vi "Outlook_Body_InsertPicture.vi"(7 "show Image in the Attachments? (F)":bool, 8 "error in (no error)":errorcluster, 9 "FilePath":path, 11 "Attachment Refnum (In)":refnum<k7>) -> (0 "error out":errorcluster, 1 "PathName":string, 2 "FileName":string, 3 "Attachment Refnum (Out)":refnum<k7>, 4 "DisplayName":string, 6 "Class":i32)   [LabVIEW 2014]
panel:
  out "Size":i32
  out "Position":i32
  out "Type":i32
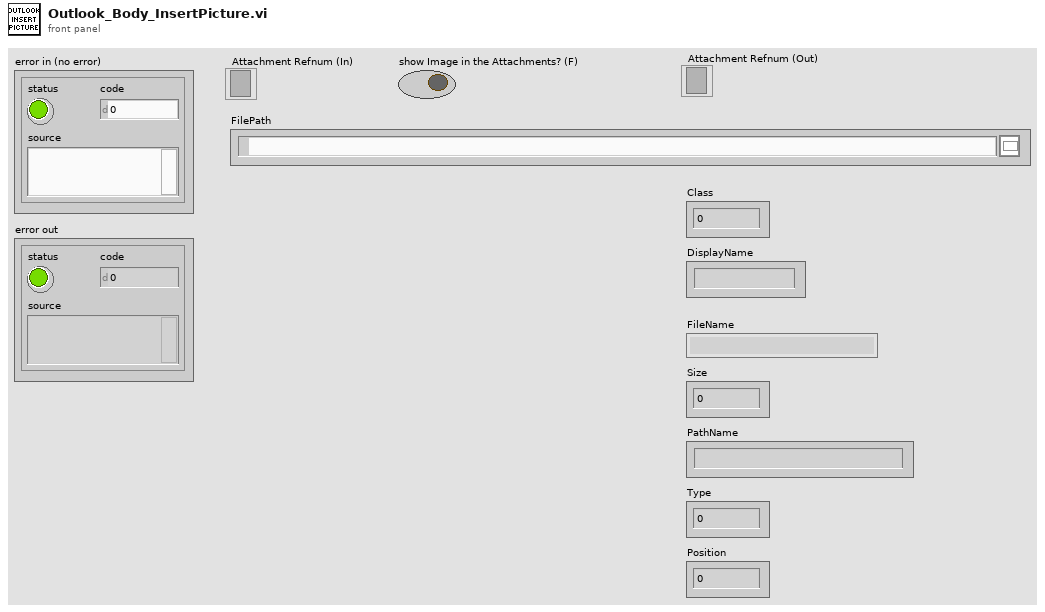
[diagram p1: front panel]
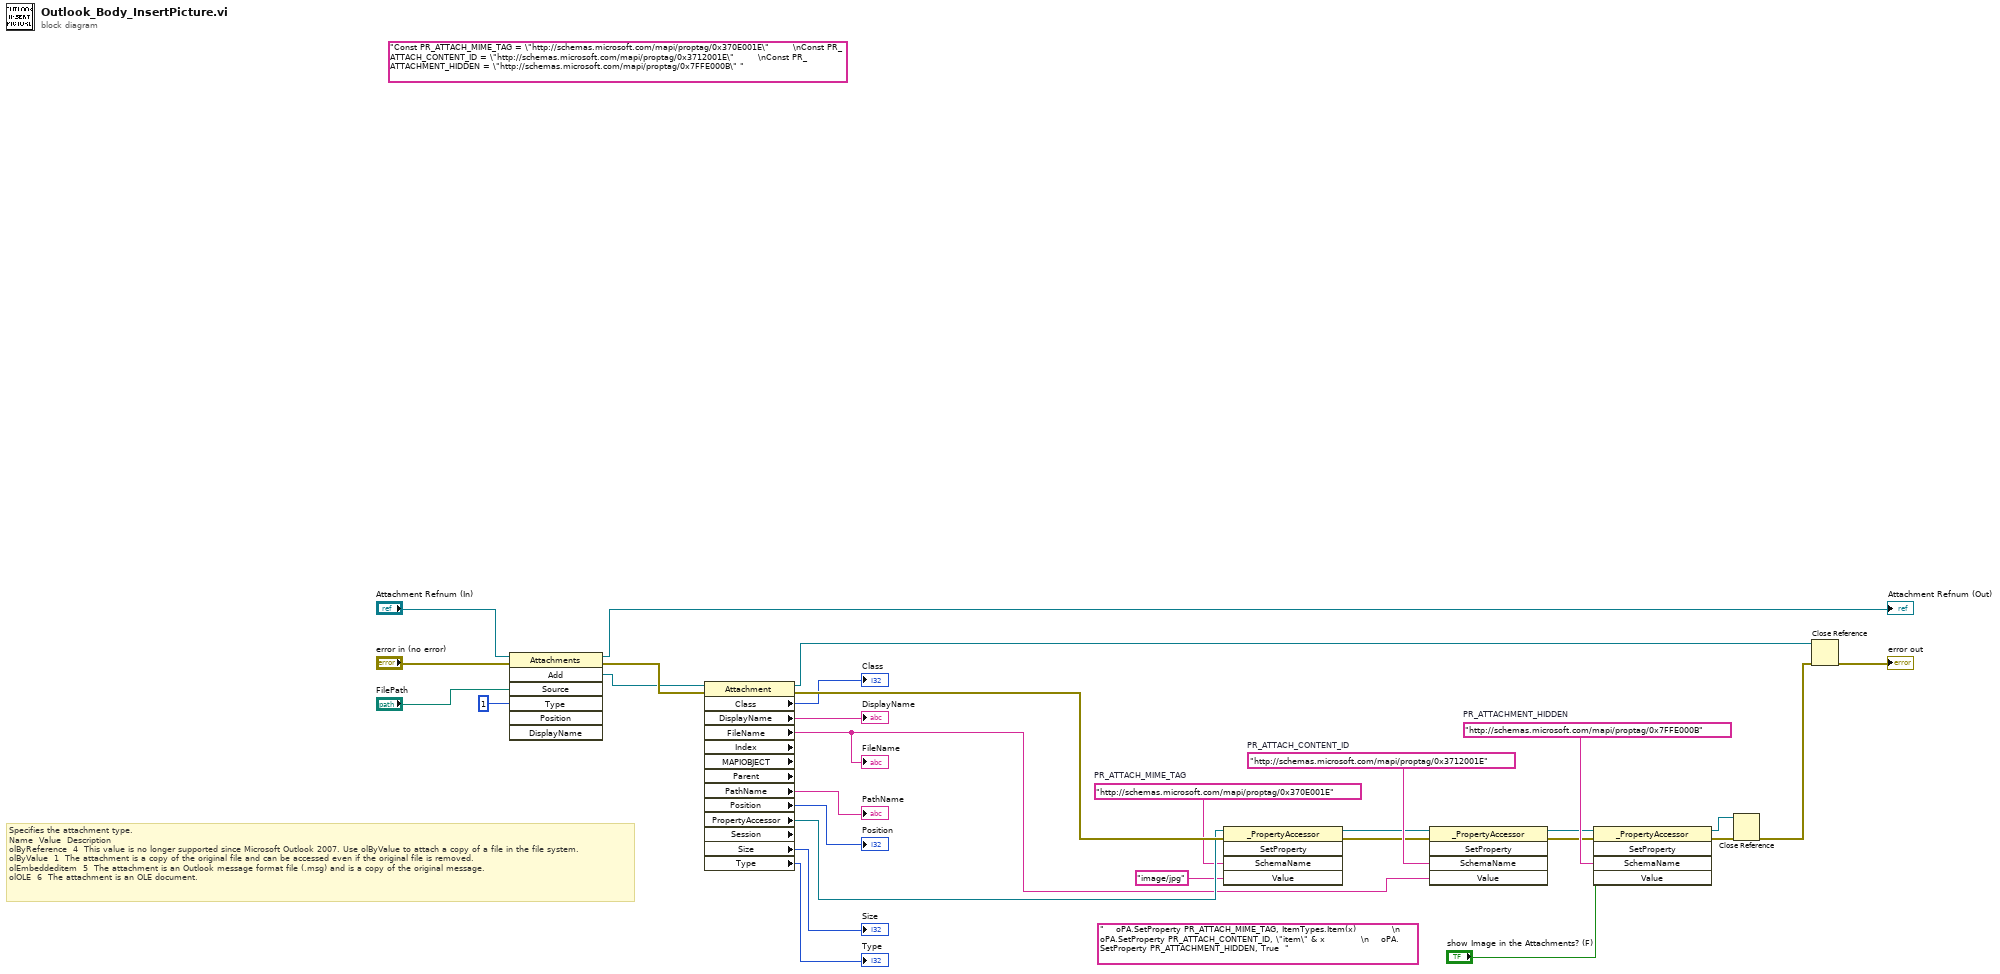
[diagram p0: block diagram]
diagram:
  w24 = "http://schemas.microsoft.com/mapi/proptag/0x7FFE000B"  # PR_ATTACHMENT_HIDDEN
  w23 = "http://schemas.microsoft.com/mapi/proptag/0x3712001E"  # PR_ATTACH_CONTENT_ID
  w18 = "http://schemas.microsoft.com/mapi/proptag/0x370E001E"  # PR_ATTACH_MIME_TAG
  (unwired) "Const PR_ATTACH_MIME_TAG = \"http://schemas.microsoft.com/mapi/proptag/0x370E001E\"        \nConst PR_ATTACH_CONTENT_ID = \"http://schemas.microsoft.com/mapi/proptag/0x3712001E\"        \nConst PR_ATTACHMENT_HIDDEN = \"http://schemas.microsoft.com/mapi/proptag/0x7FFE000B\" "
  (unwired) "    oPA.SetProperty PR_ATTACH_MIME_TAG, ItemTypes.Item(x)            \n    oPA.SetProperty PR_ATTACH_CONTENT_ID, \"item\" & x            \n    oPA.SetProperty PR_ATTACHMENT_HIDDEN, True  "
  # "Specifies the attachment type.\nName \tValue \tDescription\nolByReference \t4 \tThis value is no longer supported since Microsoft Outlook 2007. Use olByValue to attach a copy of a file in the file system.\nolByValue \t1 \tThe attachment is a copy of the original file and can be accessed even if the original file is removed.\nolEmbeddeditem \t5 \tThe attachment is an Outlook message format file (.msg) and is a copy of the original message.\nolOLE \t6 \tThe attachment is an OLE document."
  n1 = invoke class="Attachments" method="Add"(reference="Attachment Refnum (In)", error in="error in (no error)", "Source"="FilePath", "Type"=1) -> (reference out=→"Attachment Refnum (Out)":refnum<k7>, error out=w30:errorcluster, "Add"=w27:refnum<k7>)  [unwired: 3 in, 4 out]
  n2 = property class="Attachment" props=["Class", "DisplayName", "FileName", "Index", "MAPIOBJECT", "Parent", "PathName", "Position", "PropertyAccessor", "Session", "Size", "Type"](reference=w27, error in=w30) -> (reference out=w4:refnum<k7>, error out=w29:errorcluster, "Class"=→"Class":i32, "DisplayName"=→"DisplayName":string, "FileName"=w26:string, "PathName"=→"PathName":string, "Position"=→"Position":i32, "PropertyAccessor"=w28:refnum<k7>, "Size"=→"Size":i32, "Type"=→"Type":i32)  [unwired: 4 out]
  "FileName" <- w26
  n3 = invoke class="_PropertyAccessor" method="SetProperty"(reference=w28, error in=w29, "SchemaName"=w18, "Value"="image/jpg" ("SchemaName")) -> (reference out=w19:refnum<k7>, error out=w22:errorcluster)  [unwired: 1 in, 3 out]
  n4 = invoke class="_PropertyAccessor" method="SetProperty"(reference=w19, error in=w22, "SchemaName"=w23, "Value"=w26) -> (reference out=w20:refnum<k7>, error out=w21:errorcluster)  [unwired: 1 in, 3 out]
  n5 = invoke class="_PropertyAccessor" method="SetProperty"(reference=w20, error in=w21, "SchemaName"=w24, "Value"="show Image in the Attachments? (F)") -> (reference out=w5:refnum<k7>, error out=w6:errorcluster)  [unwired: 1 in, 3 out]
  n6 = Close Reference(reference=w5, error in (no error)=w6) -> (error out=w2:errorcluster)
  n7 = Close Reference(reference=w4, error in (no error)=w2) -> (error out=→"error out":errorcluster)
